vi "PDF_Interface_PDF Protokoll EPA1065_307.vi"(2 "ResultPictures":T1, 3 "PDF Optinen":T8, 4 "Deckblatt_Name":string, 5 "start":bool, 6 "SpanComponentInfos-Cluster":T7, 7 "Save PDF File Path":path, 8 "error in (no error)":errorcluster caption="Fehler (Eingang, kein Fehler)", 9 "Context (Eingang)":refnum<class "Context.lvclass">, 10 "EPA Optionsfeld":T2=enum."Rohwert", 11 "XY-Graph EPA":refnum<vi>) -> (0 "error out":errorcluster caption="Fehler (Ausgang)", 1 "Context (Ausgang)":refnum<class "Context.lvclass">)   [LabVIEW 2020, in "Linearisierung v2.lvlib" / "Protokoll.lvlib"]
uses:
  Protokoll.lvlib
  EPA Ausgabetabelle.ctl
  AktivArray.ctl
  AktivButton.ctl
  <vilib>/Simplicity AI/SAI_PDF_API/Classes/Context/Context.lvclass
  SpanEinstellungen/PDF Optionen.ctl
  SpanEinstellungen/SpanComponentInfos-Cluster.ctl
  SpanEinstellungen/ComponentInfos.ctl
  Visualisierungs Elemente/String - Ausgabefeld.ctl
  Visualisierungs Elemente/String - Eingabefeld.ctl
  EPA Optionsfeld.ctl
  PDF_Interface/PDF Interface Helper/PDFResultPictures.ctl
  Sprachverwaltung/FGV Aktion Tabelle zerlegen.ctl
  Aktion Lin Daten aufarbeiten.ctl
  EPA1065-307/Aktion FGV Auswertung sammeln.ctl
  Seiten/FT-IR/FGV FT-IR Aktionen.ctl
  Seiten/System Einstellungen V2/Aktioen FGV System Konstanten.ctl
  Seiten/FT-IR/FGV FT-IR Gasliste Aktionen.ctl
  Seiten/System Einstellungen V2/Aktion FGV SystemEinstellungenV2.ctl
  Gasteiler/Aktionen FGV Gasteiler Daten.ctl
  PDF_Interface/PDF Protokoll Standard Kopf Optionen.ctl
  PDF_Interface/PDF Interface Helper/PDFGraph.ctl
  <vilib>/Simplicity AI/SAI_PDF_API/Classes/Context/Controls/SAI_PDF_Text Align.ctl
  PDF_Interface/PDF Interface Helper/PDFCommentPosition.ctl
  PDF_Interface/PDF Interface Helper/PDFPageBreak.ctl
  <vilib>/Simplicity AI/SAI_PDF_API/Classes/Context/Controls/SAI_PDF_PDF Details.ctl
  PDF_Interface/PDF Interface Helper/PDFContentType.ctl
  PDF_Interface/PDF Interface Helper/PDFTableContentType.ctl
  PDF_Interface/PDF Interface Helper/PDFResults.ctl
  PDF_Interface/PDF Interface Helper/PDFTablePictures.ctl
  PDF_Interface/PDF Interface Helper/PDFBemerkung.ctl
  <vilib>/Simplicity AI/SAI_PDF_API/Classes/Context/Controls/SAI_PDF_Font.ctl
  <vilib>/Simplicity AI/SAI_PDF_API/Classes/Context/Controls/SAI_PDF_Font Encoding.ctl
  PDF_Interface/PDF Interface Helper/PDFTtilePageContentType.ctl
  Gasteiler/HovaCAL_Interface/Kommunikation/Aktion FGV HovaCAL Interface Autolin.ctl
  GasteilerType.ctl
  Linearisierung v2.lvlib
  EPA1065-307/Linearity verification 1065-307.lvlib
  Allgemein/allgemeine Sub-VIs.lvlib
  Seiten/FT-IR/FT-IR.lvlib
  Seiten/System Einstellungen V2/System Einstellungen V2.lvlib
  Gasteiler/Gasteiler.lvlib
  PDF_Interface/PDF Interface.lvlib
  Sprachverwaltung/Sprachverwaltung.lvlib
  PDF_Interface/PDF Interface Helper/PDF Interface Helper.lvlib
  Gasteiler/HovaCAL_Interface/Kommunikation/Kommunikation.lvlib
  SpanEinstellungen/SpanEinstellungen.lvlib
panel:
  out "Messwert:":string
  out "Serial number GT":string caption="Seriennummer:"
  out "Accuracy:":string caption="Genauigkeit:"
  out "Gas Bottle Nr.:":string caption="Gasflaschen Nr.:"
  out "Methode (Recipe):":string caption="Methode (Rezept):"
  out "Date & Time:":string caption="Datum & Zeit:"
  out "Versa Serial number:":string caption="Seriennummer:"
  out "Anlage:":string
  out "Serial number:":string caption="Seriennummer:"
  out "Messgerät:":string
  out "XY-Graph EPA":cluster{dbl[], dbl[]}[](graph) caption="XY-Graph"
  out "Aktiv":T9
  out "EPA Ausgabetabelle":T11
  out "Ergebnis:":string
  out "Konzentration:":string
  out "Komponente:":string
  out "Bearbeiter:":string
  out "Gasteiler:":string
  out "EPA Auswertung":string[][](table) caption="Evaluation"
  # "Linearity Check EPA § 1065.307"
  # "Linearity detection §1065.307"
  # "Description of the limits"
  # "Slope (a1) value between 0,99-1,01"
  # "Intercept (a0)"
  # "laboratory: Value <= 0,5% of the gas concentration"
  # "field: Value <= 1% of the gas concentration"
  # "Coefficient of determination (R²) Value >= 0,998"
  # "standard error of estimate (SEE) Value <= 1% of the gas concentration"
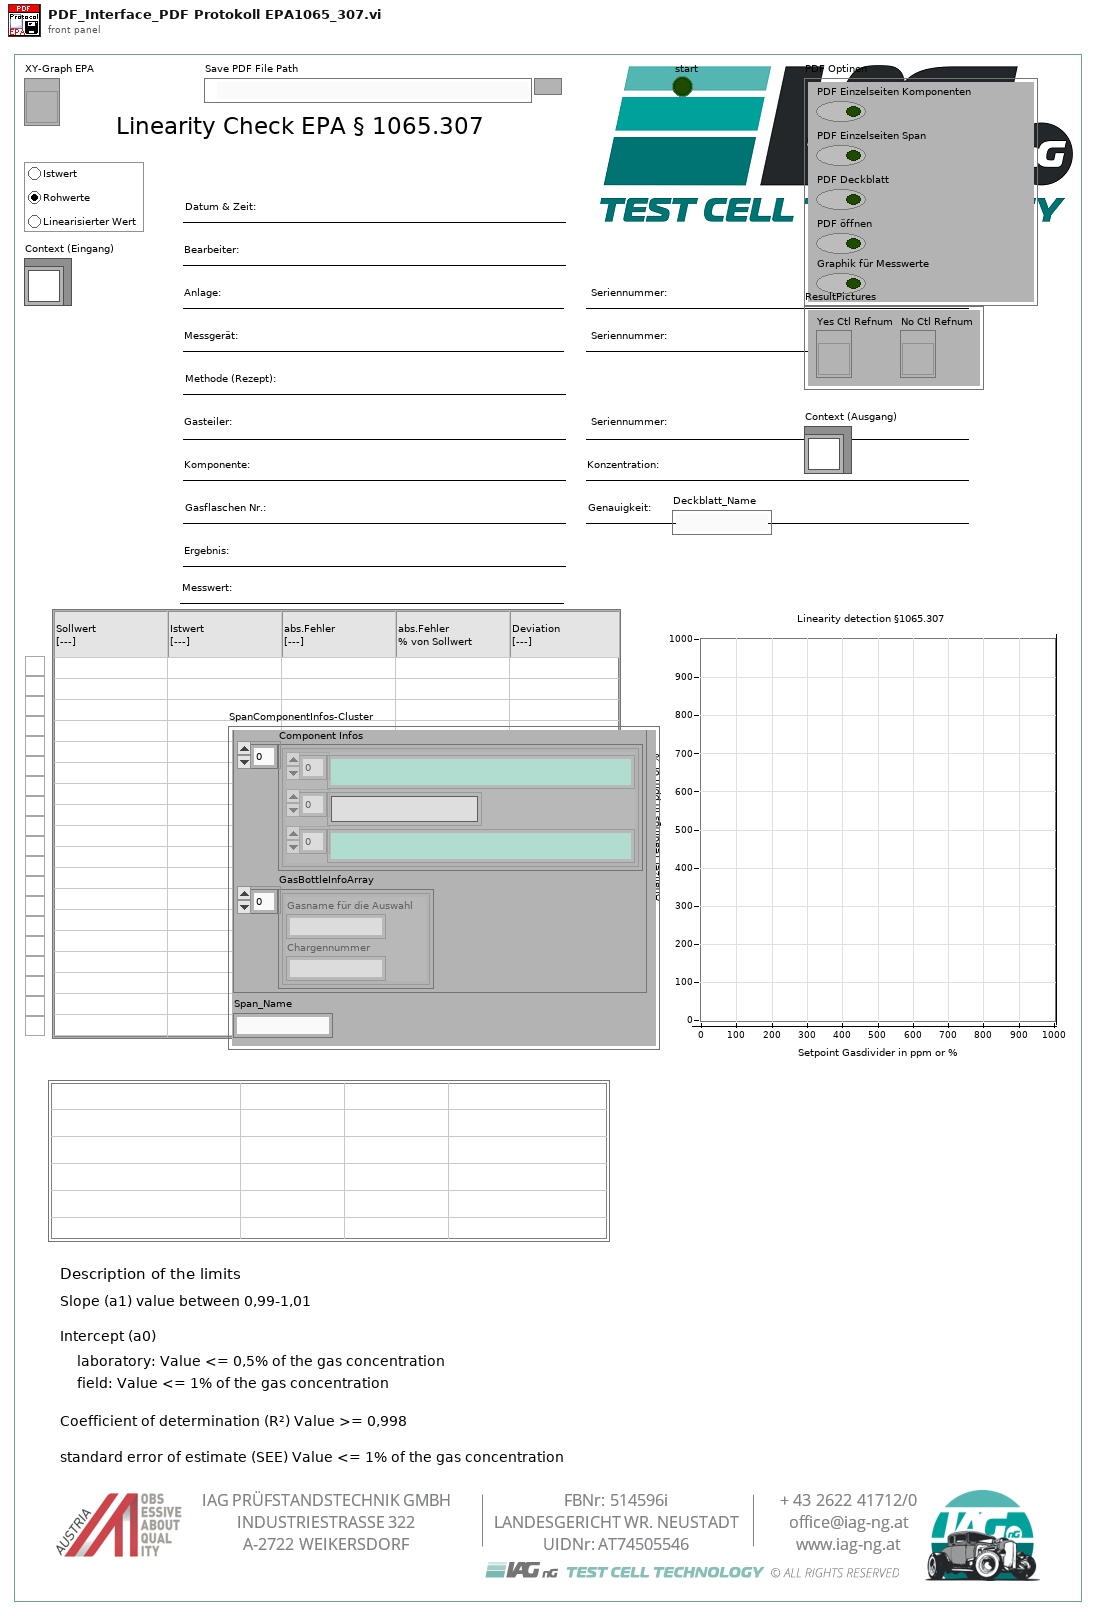
[diagram p1: front panel]
types:
  T1 = typedef "PDF Interface.lvlib/PDF Interface Helper.lvlib/PDFResultPictures.ctl" = cluster{"Yes Ctl Refnum":refnum<vi>, "No Ctl Refnum":refnum<vi>}
  T2 = typedef "Linearisierung v2.lvlib/EPA Optionsfeld.ctl" = enum32{"Istwert", "Rohwert", "Linearisierter Wert"}
  T3 = typedef "Linearisierung v2.lvlib/SpanEinstellungen.lvlib/SpanComponentInfos-Cluster.ctl" = cluster{"SPAN Names":string[], "Component Infos":T4[], "GasBottleInfoArray":cluster{"Gasname für die Auswahl":string, "Chargennummer":string}[]}
  T4 = typedef "Linearisierung v2.lvlib/SpanEinstellungen.lvlib/ComponentInfos.ctl" = cluster{T5[], T6[], T5[]}
  T5 = typedef "String - Ausgabefeld.ctl" = string
  T6 = typedef "String - Eingabefeld.ctl" = string
  T7 = cluster{"SpanComponentInfos-Cluster":T3, "Span_Name":string}
  T8 = typedef "Linearisierung v2.lvlib/SpanEinstellungen.lvlib/PDF Optionen.ctl" = cluster{"PDF Einzelseiten Komponenten":bool, "PDF Einzelseiten Span":bool, "PDF Deckblatt":bool, "PDF öffnen":bool, "Graphik für Messwerte":bool}
  T9 = typedef "Linearisierung v2.lvlib/AktivArray.ctl" = T10[]
  T10 = typedef "Linearisierung v2.lvlib/AktivButton.ctl" = bool
  T11 = typedef "Linearisierung v2.lvlib/EPA Ausgabetabelle.ctl" = string[][]
  T12 = typedef "Sprachverwaltung.lvlib/FGV Aktion Tabelle zerlegen.ctl" = enum16{"laden", "vereinzeln", "speichern"}
  T13 = typedef "PDF Interface.lvlib/PDF Protokoll Standard Kopf Optionen.ctl" = cluster{"Analysator":bool, "FT-IR Rezept":bool, "Gasteiler":bool, "Gas Komponente":bool, "Gas Flasche":bool, "LIN Protokoll":bool, "Operator":bool}
  T14 = typedef "Linearisierung v2.lvlib/Gasteiler.lvlib/Aktionen FGV Gasteiler Daten.ctl" = enum16{"lesen", "Gasteiler Daten", "Seriellen Param.", "MB-Endwert", "laden", "speichern", "Anforderung", "TCP", "Aufzeichnung Start"}
  T15 = typedef "System Einstellungen V2.lvlib/Aktion FGV SystemEinstellungenV2.ctl" = enum16{"lesen", "Analysatoren schreiben", "Analysator ändern", "Analysatoren löschen", "laden", "speichern", "Untertitel", "Analysatoren", "Neue Analysatoren", "Gasteiler schreiben", "Gasteiler ändern", "Gasteiler löschen", "Gasteiler", "Gasteiler exportieren", "Gasteiler importieren"}
  T16 = typedef "FT-IR.lvlib/FGV FT-IR Gasliste Aktionen.ctl" = enum16{"lesen", "Gasliste FT-IR", "Gasliste ausgelesen", "laden", "speichern", "löschen"}
  T17 = typedef "System Einstellungen V2.lvlib/Aktioen FGV System Konstanten.ctl" = enum16{"lesen", "laden", "speichern", "Sprache"}
  T18 = typedef "FT-IR.lvlib/FGV FT-IR Aktionen.ctl" = enum16{"lesen", "NOG setzen", "NOS setzen", "Initialisieren", "speichern", "ALLES setzen", "FT-IR Spektrum loggen", "Komm Stoppen", "Spektrum LogKonfig"}
  T19 = typedef "Linearisierung v2.lvlib/Aktion Lin Daten aufarbeiten.ctl" = enum16{"lesen", "Protkolldaten", "speichern", "laden", "EPA auswerten", "Tabelle schreiben", "Lin auswerten", "Tab init", "Stufentabelle", "EPA aktiviert", "Nachbehandlung laden", "Tabelle löschen", "Istwerte löschen", "Zeile löschen", "Zeile einfügen", "LIN aktiviert", "LIN/EPA aktiv laden", "EGAK Tab", "LIN übernehmen", "Tab init ohne Stufen"}
  T20 = typedef "Linearisierung v2.lvlib/Linearity verification 1065-307.lvlib/Aktion FGV Auswertung sammeln.ctl" = enum16{"lesen", "Auswertung", "löschen"}
  T21 = typedef "Linearisierung v2.lvlib/Gasteiler.lvlib/HovaCAL_Interface.lvlib/Kommunikation.lvlib/Aktion FGV HovaCAL Interface Autolin.ctl" = enum16{"lesen", "schreiben", "MFC Komponente fix setzen", "init"}
  T22 = typedef "PDF Interface.lvlib/PDF Interface Helper.lvlib/PDFTableContentType.ctl" = cluster{"TableHeader":string[], "Table":string[][], "Relative Column Widths (%)":sgl[], "Results":T23, "PositionBemerkung":T24, "PageBreak":T25, "TablePictures":T26, "Horizontal Align":i32}
  T23 = typedef "PDF Interface.lvlib/PDF Interface Helper.lvlib/PDFResults.ctl" = cluster{"Results":cluster{"Result Text":string, "Result":bool}[], "ResultPictures":T1, "use Pictures":bool, "Image Scale (%)":sgl, "Autoscale? (T)":bool, "Horizontal Align":i32, "Position":i32}
  T24 = typedef "PDF Interface.lvlib/PDF Interface Helper.lvlib/PDFCommentPosition.ctl" = enum16{"before", "after"}
  T25 = typedef "PDF Interface.lvlib/PDF Interface Helper.lvlib/PDFPageBreak.ctl" = enum16{"none", "before", "after", "after comment"}
  T26 = typedef "PDF Interface.lvlib/PDF Interface Helper.lvlib/PDFTablePictures.ctl" = cluster{"Ctl Refnum In":refnum<vi>[], "RowOrColumn":enum16{"Row", "Column"}, "IndexToInsert":u16, "Image Scale (%)":sgl[], "Autoscale? (T)":bool[], "Horizontal Align":i32}
  T27 = typedef "SAI_PDF_Toolkit.lvlib/Context.lvclass/SAI_PDF_Font.ctl" = cluster{"Font":string, "Size":i32, "Colour":u32, "Bold":bool, "Italic":bool, "Underline":bool, "Strikethrough":bool, "Font Encoding":T28}
  T28 = typedef "SAI_PDF_Toolkit.lvlib/Context.lvclass/SAI_PDF_Font Encoding.ctl" = enum16{"Cp1252, WinANSI", "IdentityH", "IdentityV", "Cp1250", "Cp1257", "MacRoman"}
  T29 = typedef "PDF Interface.lvlib/PDF Interface Helper.lvlib/PDFTtilePageContentType.ctl" = cluster{"Titel":string, "Header Tables":string[][][], "Bemerkungen":T30[]}
  T30 = typedef "PDF Interface.lvlib/PDF Interface Helper.lvlib/PDFBemerkung.ctl" = cluster{"Bemerkung Text":string, "Align (Left)":T31, "Add Line Feeds (F:No)":bool, "Font":T27}
  T31 = typedef "SAI_PDF_Toolkit.lvlib/Context.lvclass/SAI_PDF_Text Align.ctl" = i32
  T32 = typedef "PDF Interface.lvlib/PDF Interface Helper.lvlib/PDFGraph.ctl" = cluster{"GraphCtl Refnum":refnum<vi>, "Wrap Text (F:No)":bool, "Hide Grid (F:No)":bool, "Scale (100%)":sgl, "Align (Left)":T31, "PositionBemerkung":T24, "PageBreak":T25}
  T33 = typedef "PDF Interface.lvlib/PDF Interface Helper.lvlib/PDFContentType.ctl" = cluster{"Titel":string, "Header Table":string[][], "Table Array":T22[], "Bemerkungen":T30[]}
  T34 = typedef "SAI_PDF_Toolkit.lvlib/Context.lvclass/SAI_PDF_PDF Details.ctl" = cluster{"Title":string, "Subject":string, "Keywords":string, "Author":string, "Creator":string}
  T35 = cluster{"Header Footer Text Cluster":cluster{"Header Text":string, "Footer Text":string, "Time":string, "Page Number":string}, "PDF Details":T34}
  T36 = typedef "System Einstellungen V2.lvlib/Gasteiler.ctl" = cluster{"Gasteiler Name":string, "Gasteiler Type":string, "Gasteiler Seriennummer":string, "Gasteiler Letzte Wartung":timestamp}
  T37 = cluster{"GasteilerDefinitionsListe":T36[], "GasteilerDefinitionTextliste":string[][], "Gasteiler Strings And Values":cluster{"String":string, "Wert":string}[]}
  T38 = typedef "Linearisierung v2.lvlib/Gasteiler.lvlib/Gasteiler Daten.ctl" = cluster{"Gasteiler":T6, "Gasteiler Stufen":T39, "Gasteiler Type":T40, "Konfig Gasteiler":T41, "Gasteiler Span Eingänge":u16}
  T39 = typedef "Linearisierung v2.lvlib/Gasteiler.lvlib/Gasteiler Stufen.ctl" = u16
  T40 = typedef "Linearisierung v2.lvlib/GasteilerType.ctl" = u16
  T41 = typedef "System Einstellungen V2.lvlib/Gasteiler Auswahl.ctl" = u16
  T42 = cluster{"Modell":string, "ProjektNummer":string, "Software Version":string, "Seriennummer":string}
  T43 = typedef "Auswahlfeld.ctl" = u16
  T44 = typedef "Linearisierung v2.lvlib/Eingabetabelle.ctl" = string[][]
  T45 = typedef "Linearisierung v2.lvlib/Lin-Polynom Daten.ctl" = cluster{"Messgerät":string, "Kalibrator (Gasteiler)":string, "Bearbeiter/in":string, "Komponente":string, "Zeitstempel":timestamp, "F_max gefordert (%)":sgl, "F_max in %":sgl, "F_max in ppm":sgl, "Vorschlag Ordnung":i32, "Polynom OK":bool, "Polynomkoeff.":dbl[], "Prüfgas Konzentration":dbl, "Pfad EPA":string, "Pfad_LIN":string, "Gasnummer:":u8, "Komponentenauswahl":T46, "Verdünnungsgas":T47, "Zeitdauer Stufe":T48, "Anzahl Stufen":T48, "F_max in % EPA":sgl, "F_max in ppm EPA":sgl, "F_max in % LIN":sgl, "F_max in ppm LIN":sgl, "Punkte umkehren":bool, "EPA Optionsfeld":T2, "Autolin Hovacal":T49, "Spanfactors":sgl[], "Kalibrierauswahl":T50, "Conditions:":T51, "Gasflaschen Nr.:":string, "Bottle Accuracy":dbl, "Konfig Gasflasche":T52, "Gasflasche":T53, "HovaCAL Flow AutoLin":T54, "MFC Output":T55, "Gas Ablaufdatum":timestamp, "Lin Modus":T56, "zusätzliche Zeitdauer Erster Punkt":sgl, "Offsets":sgl[]}
  T46 = typedef "Linearisierung v2.lvlib/KomponentenArray.ctl" = cluster{"Komponente:":T43, "Konzentration":dbl}[]
  T47 = typedef "Linearisierung v2.lvlib/Gasteiler.lvlib/Prüfgas in.ctl" = u16
  T48 = typedef "Zahlen-Eingabefeld.ctl" = sgl
  T49 = typedef "Linearisierung v2.lvlib/Gasteiler.lvlib/HovaCal.lvlib/AutoLin Hovacal.ctl" = enum32{"Keine Auswahl", "Optionsauswahl 1", "Optionsauswahl 2"}
  T50 = typedef "Linearisierung v2.lvlib/Kalibrieroption.ctl" = u16
  T51 = typedef "Linearisierung v2.lvlib/Linearity verification 1065-307.lvlib/Condition.ctl" = u16
  T52 = typedef "System Einstellungen V2.lvlib/Konfig Gasflasche.ctl" = bool
  T53 = typedef "System Einstellungen V2.lvlib/Gasflasche Auswahl.ctl" = u16
  T54 = typedef "Linearisierung v2.lvlib/Gasteiler.lvlib/HovaCAL_Interface.lvlib/Controls.lvlib/Flow Einstellung.ctl" = cluster{"HovaCAL Flow Input Cluster":dbl}
  T55 = typedef "Linearisierung v2.lvlib/Gasteiler.lvlib/HovaCAL_Interface.lvlib/Controls.lvlib/Pump state.ctl" = cluster{"Run":bool}
  T56 = typedef "CalGas Aufschaltung.lvlib/Lin Modus.ctl" = u16
  T57 = cluster{"Header Size":i32, "Column Ratio left":sgl[]}
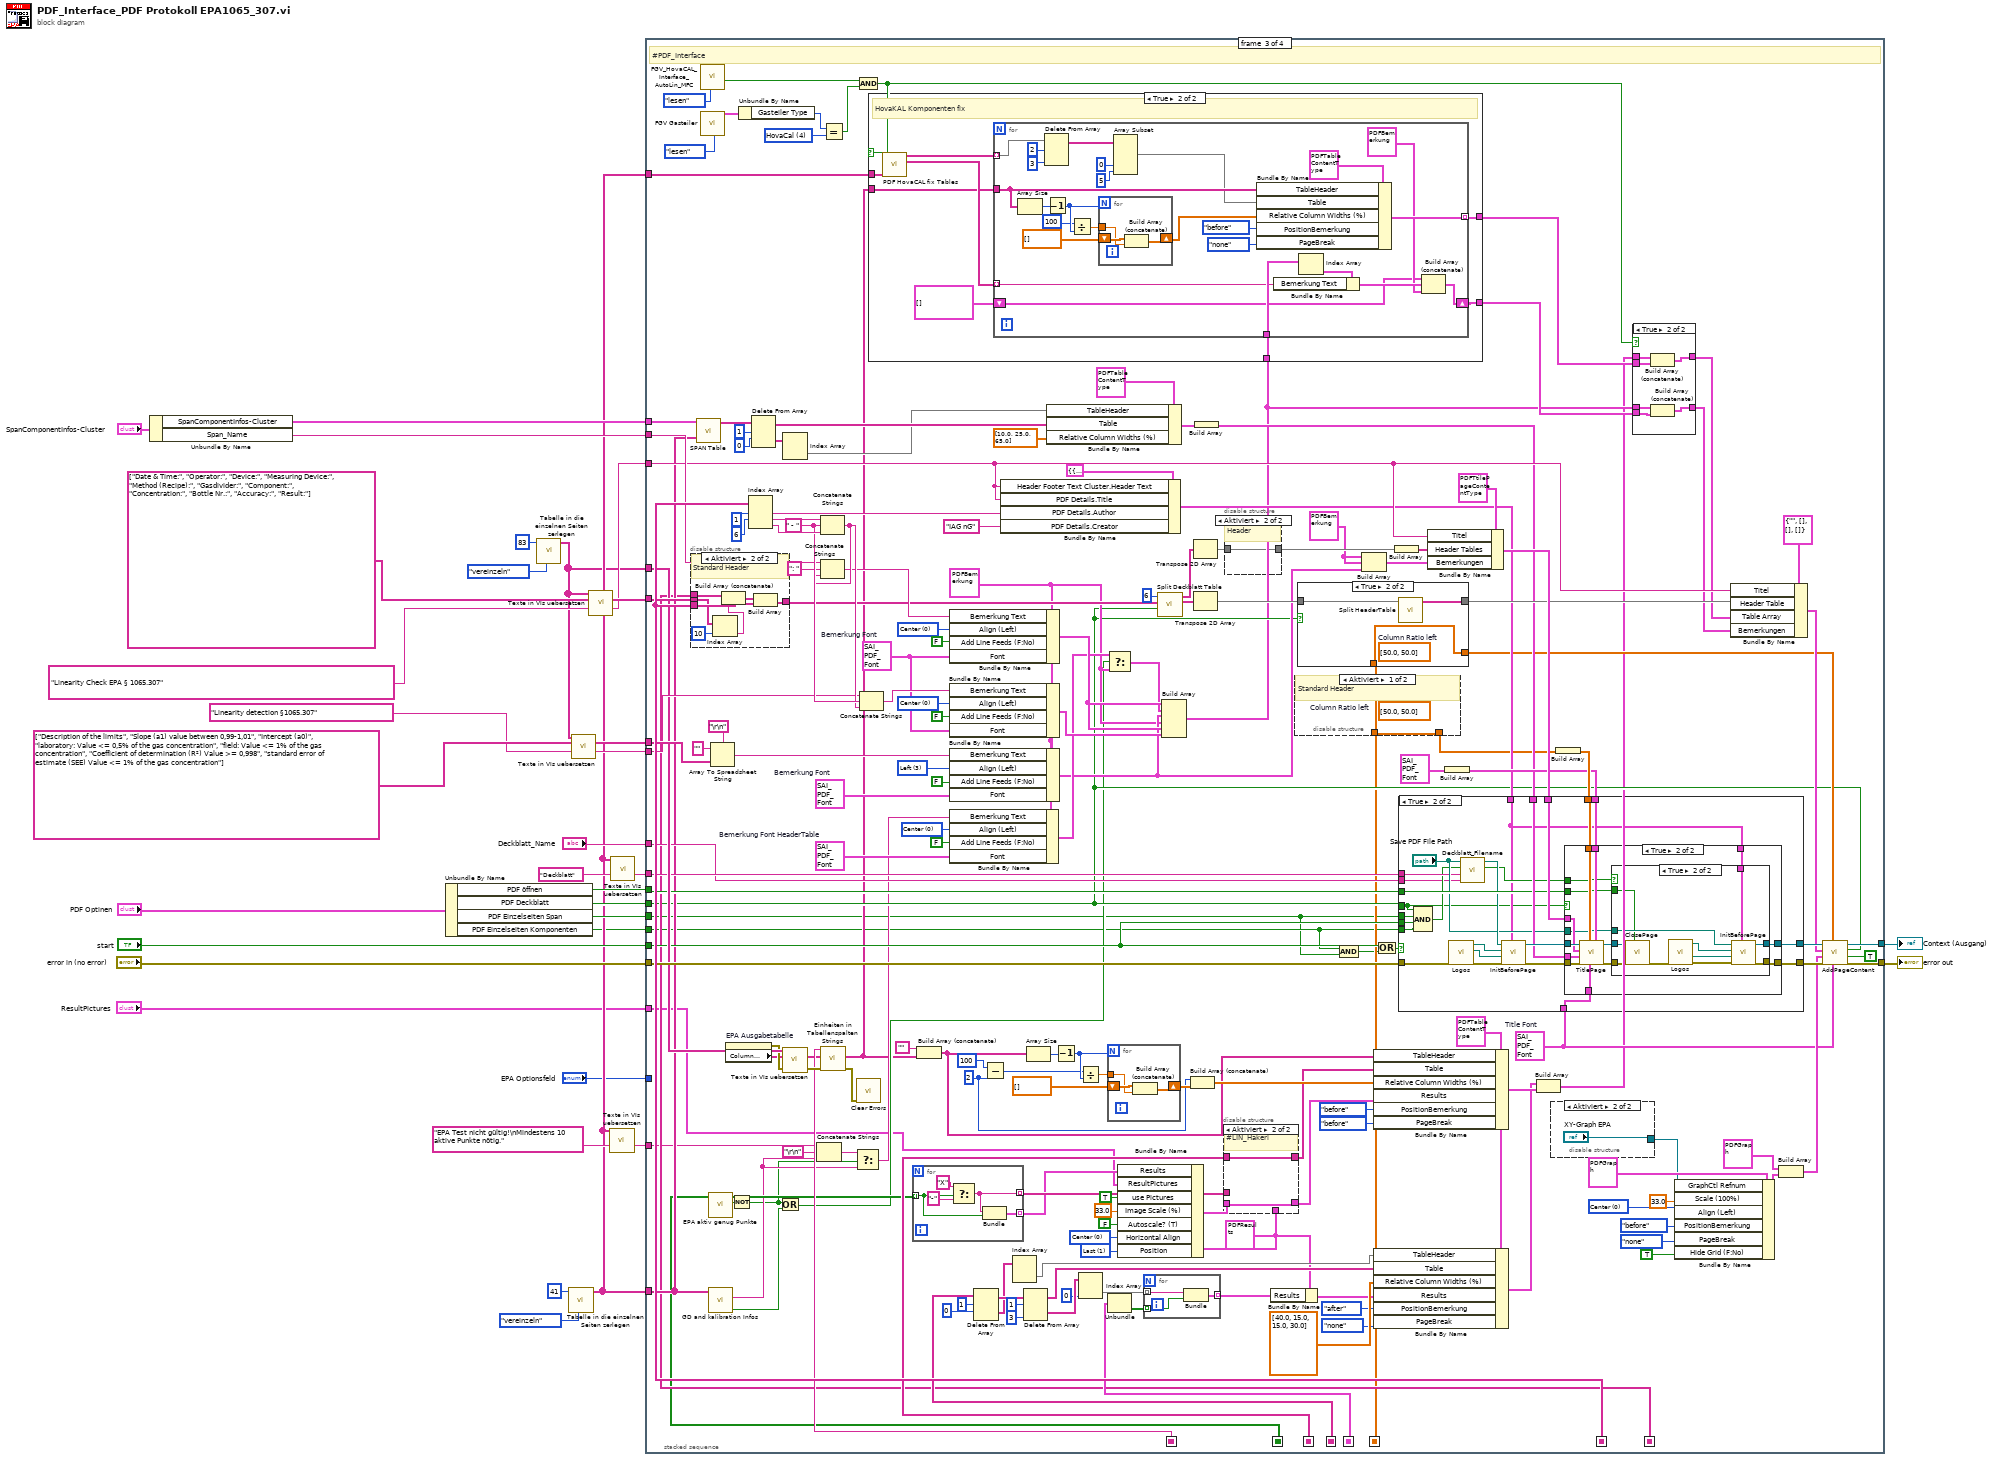
[diagram p0: block diagram]
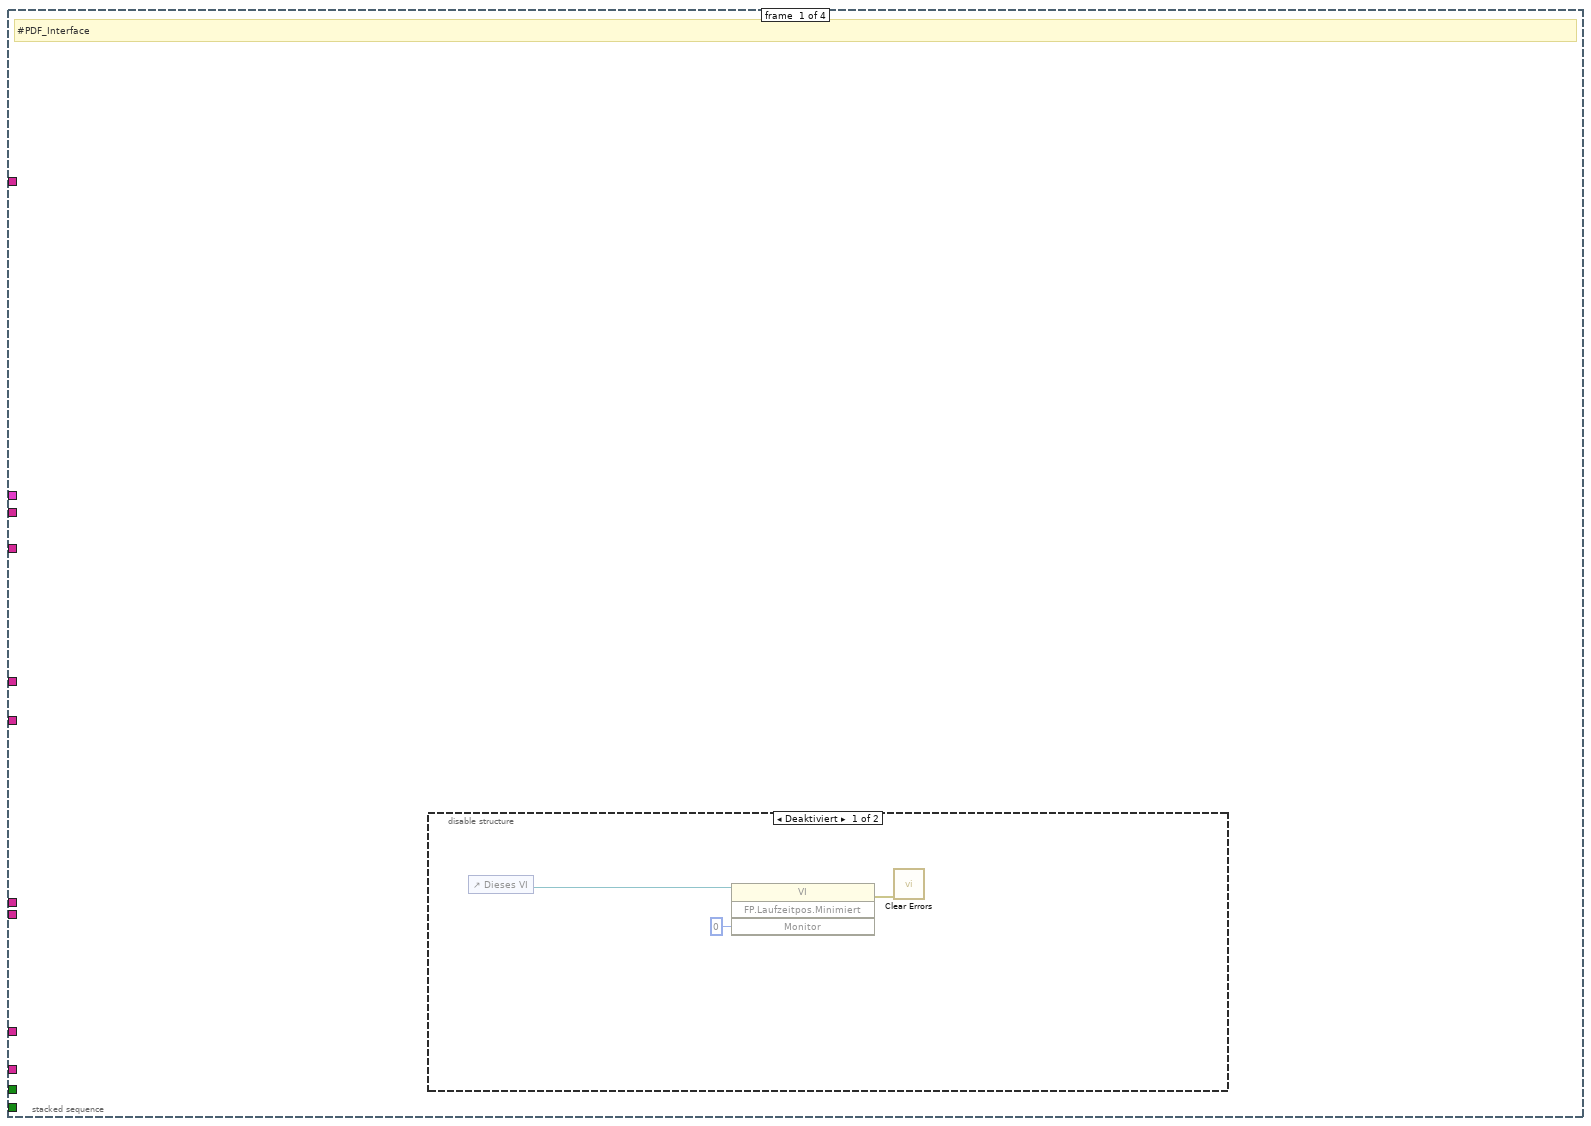
[diagram p2: hidden frame]
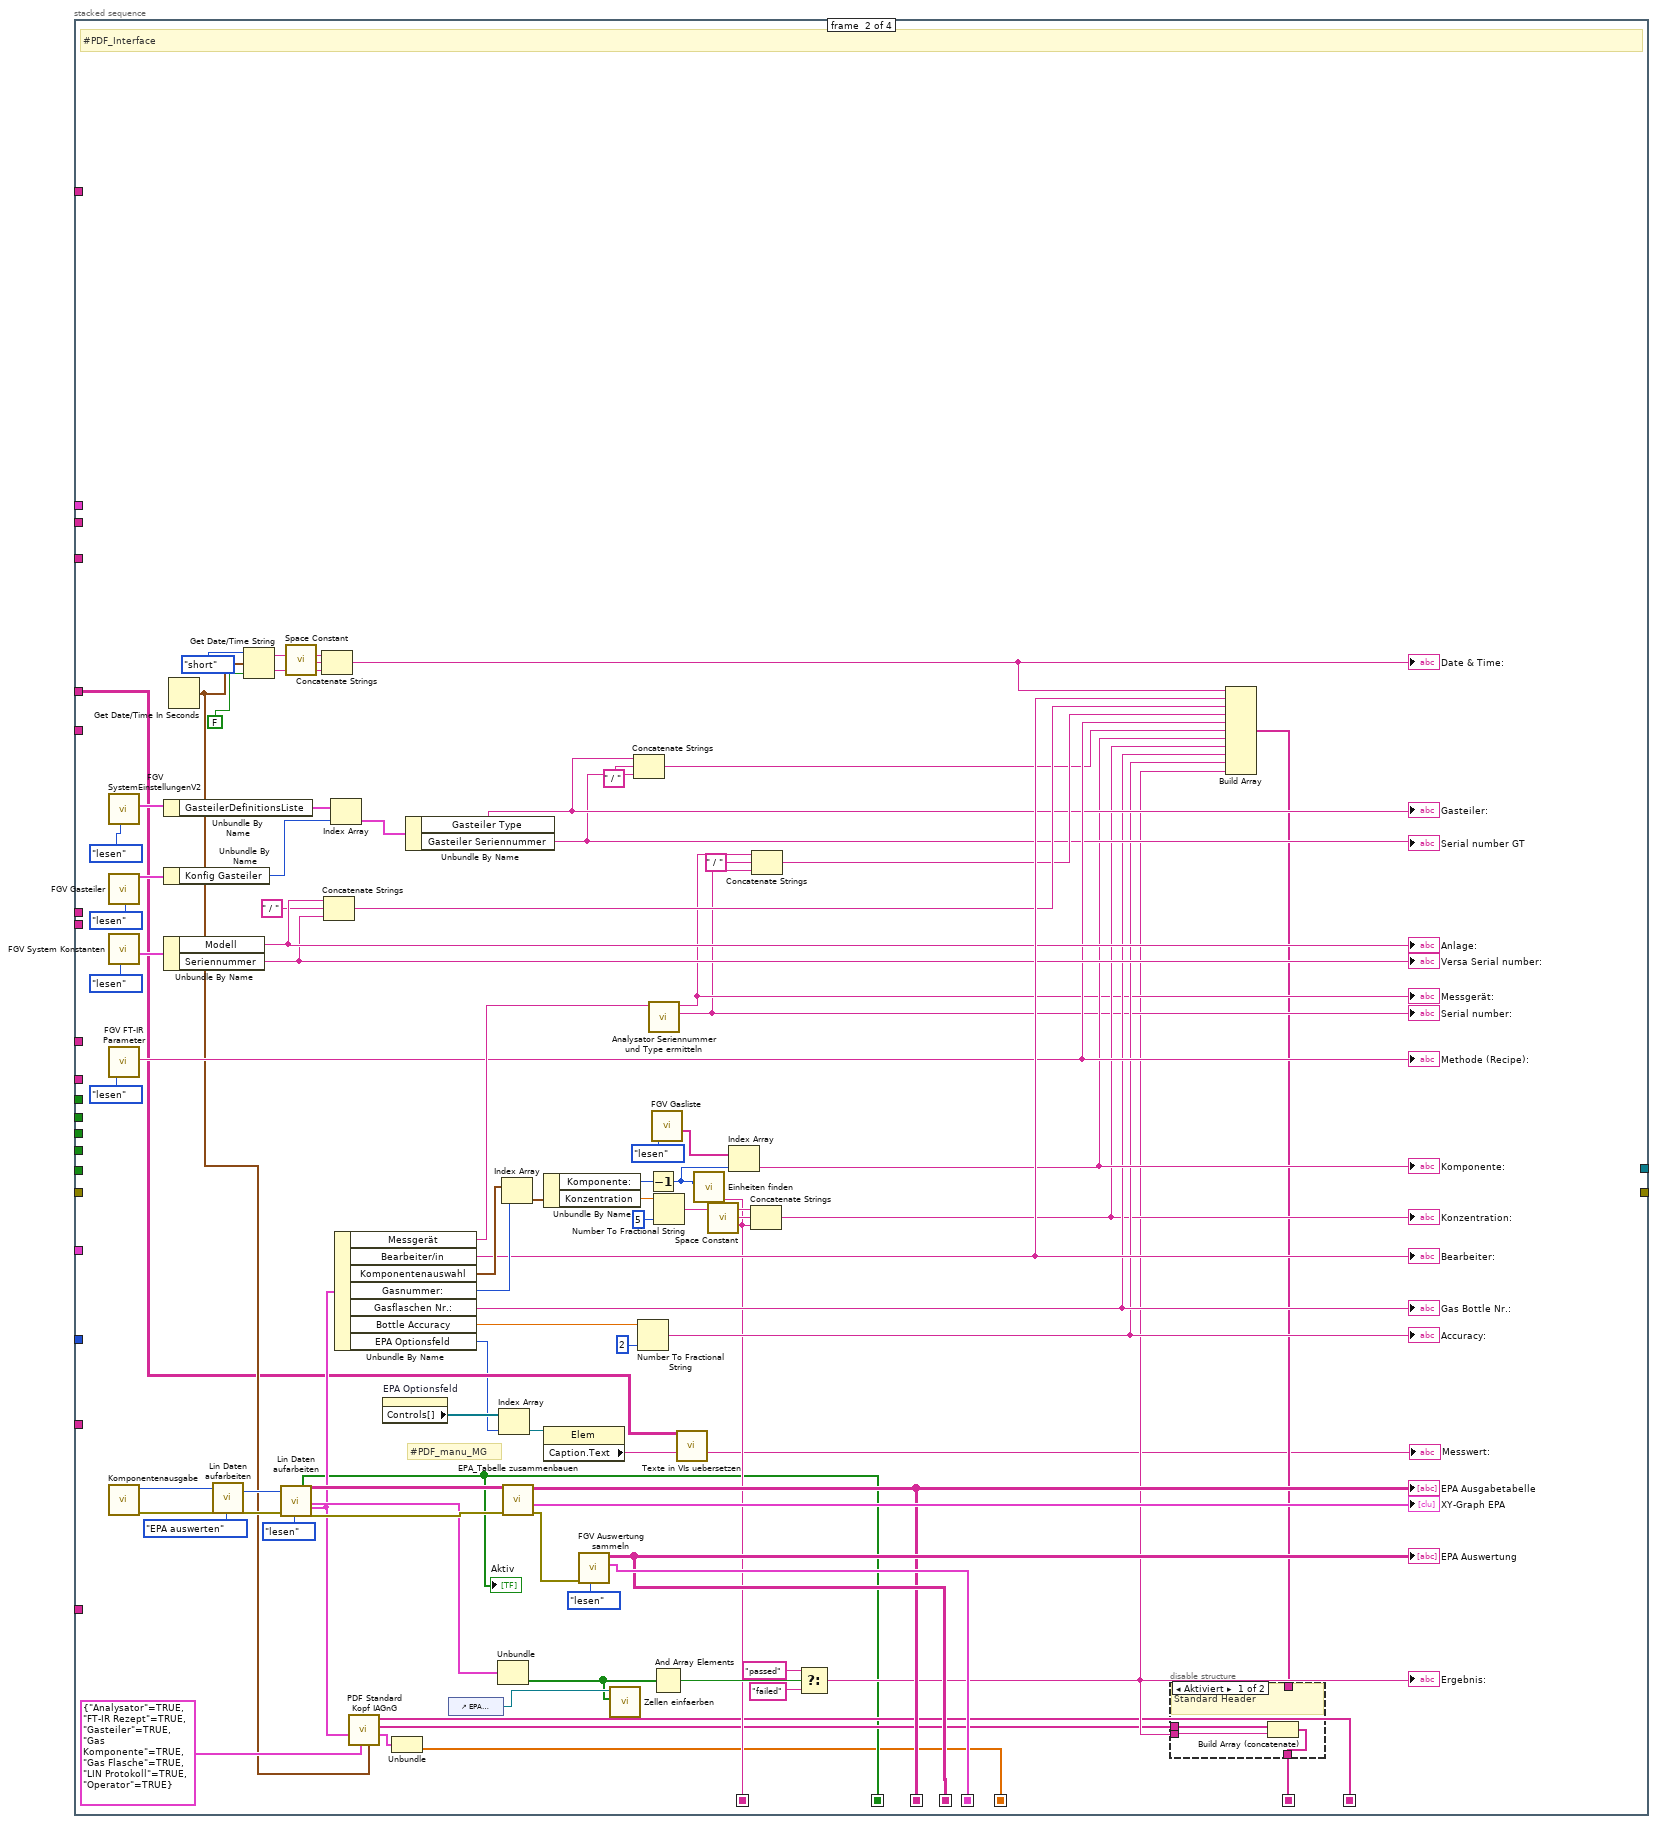
[diagram p4: hidden frame]
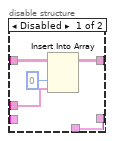
[diagram p6: hidden frame]
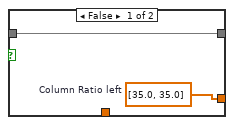
[diagram p9: hidden frame]
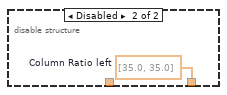
[diagram p10: hidden frame]
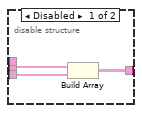
[diagram p11: hidden frame]
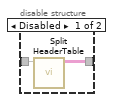
[diagram p12: hidden frame]
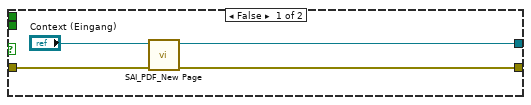
[diagram p13: hidden frame]
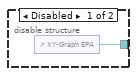
[diagram p16: hidden frame]
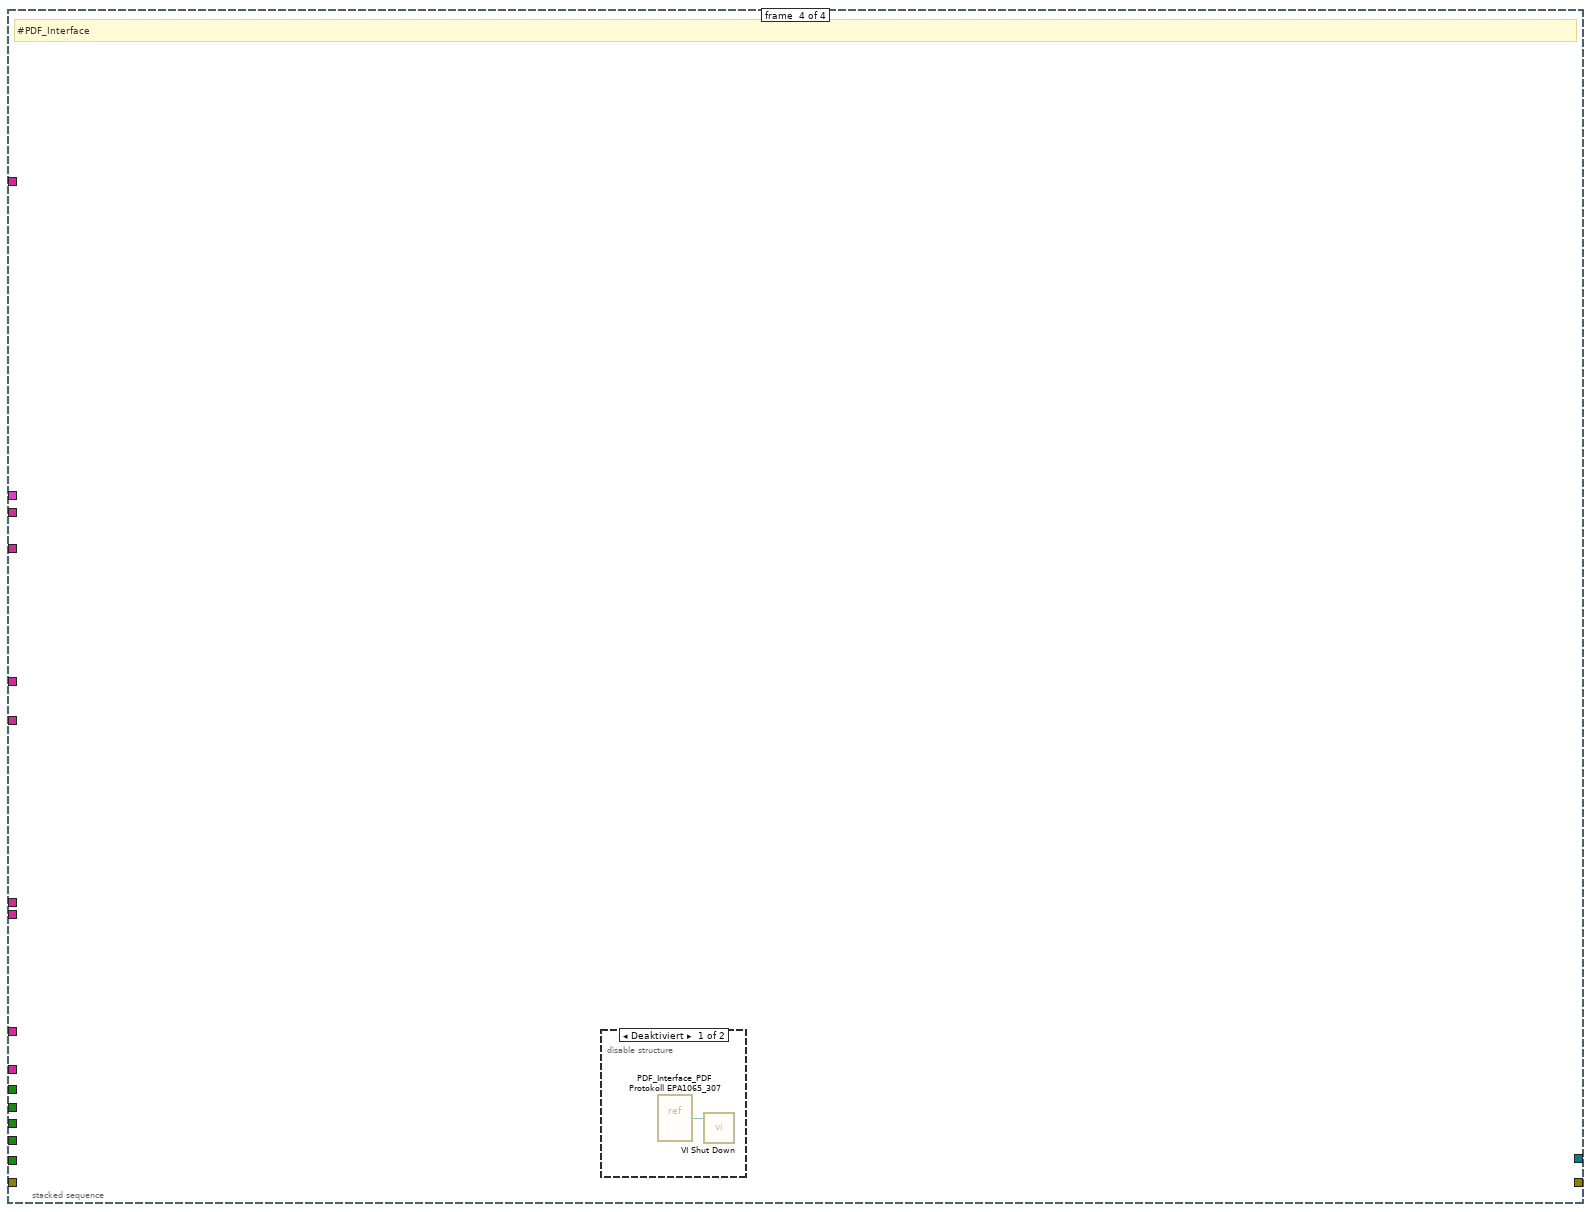
[diagram p17: hidden frame]
diagram:
  n1 = Unbundle By Name("SpanComponentInfos-Cluster") -> ("SpanComponentInfos-Cluster"=w26:T3, "Span_Name"=w29:string)
  n2 = Unbundle By Name("PDF Optinen") -> ("PDF öffnen"=w11:bool, "PDF Deckblatt"=w13:bool, "PDF Einzelseiten Span"=w12:bool, "PDF Einzelseiten Komponenten"=w2:bool)
  n3 = call "Tabelle in die einzelnen Seiten zerlegen.vi"("Aktion"=FGV_Aktion_Tabelle_zerlegen."vereinzeln", "Index (Seite)"=83) -> ("Sprachliste"=w4:string[][])  [unwired: 7 in, 2 out]
  n4 = call "Tabelle in die einzelnen Seiten zerlegen.vi"("Aktion"=FGV_Aktion_Tabelle_zerlegen."vereinzeln", "Index (Seite)"=41) -> ("Sprachliste"=w5:string[][])  [unwired: 7 in, 2 out]
  n5 = call "Texte in VIs uebersetzen.vi"("Sprachliste"=w4, "String-Array zum Übersetzen"=string[] ["Description of the limits", "Slope (a1) value between 0,99-1,01", "Intercept (a0)", "laboratory: Value <= 0,5% of the gas concentration", "field: Value <= 1% of the gas concentration", "Coefficient of determination (R²) Value >= 0,998", "standard error of estimate (SEE) Value <= 1% of the gas concentration"], "String zum Übersetzen"="Linearity detection §1065.307" ("String")) -> ("String-Array zum Übersetzen"=w17:string[], "String zum Übersetzen"=w16:string)  [unwired: 8 in, 3 out]
  n6 = call "Texte in VIs uebersetzen.vi"("Sprachliste"=w4, "String-Array zum Übersetzen"=string[] ["Date & Time:", "Operator:", "Device:", "Measuring Device:", "Method (Recipe):", "Gasdivider:", "Component:", "Concentration:", "Bottle Nr.:", "Accuracy:", "Result:"], "String zum Übersetzen"="Linearity Check EPA § 1065.307") -> ("String-Array zum Übersetzen"=w21:string[], "String zum Übersetzen"=w20:string)  [unwired: 8 in, 3 out]
  n7 = call "Texte in VIs uebersetzen.vi"("Sprachliste"=w5, "String zum Übersetzen"="EPA Test nicht gültig!\nMindestens 10 aktive Punkte nötig." ("Nachricht")) -> ("String zum Übersetzen"=w6:string)  [unwired: 9 in, 4 out]
  n8 = call "Texte in VIs uebersetzen.vi"("Sprachliste"=w5, "String zum Übersetzen"="Deckblatt") -> ("String zum Übersetzen"=w9:string)  [unwired: 9 in, 4 out]
  n9 = stacked-sequence {
    seq-local: [_ w49 _ _] -> [_ _ w296 _]
    seq-local: [_ w59 _ _] -> [_ _ w293 _]
    seq-local: [_ w64 _ _] -> [_ _ w283 _]
    seq-local: [_ w47 _ _] -> [_ _ w168 _]
    seq-local: [_ w63 _ _] -> [_ _ w281 _]
    seq-local: [_ w58 _ _] -> [_ _ w182 _]
    seq-local: [_ w48 _ _] -> [_ _ w172 _]
    seq-local: [_ w43 _ _] -> [_ _ w140 _]
    tunnel: "error in (no error)" -> [_ _ w238 _]
    tunnel: [_ _ w237 _] -> w32
    tunnel: [_ _ w236 _] -> w31
    tunnel: w29 -> [_ _ w212 _]
    tunnel: w5 -> [_ _ w174 _]
    tunnel: w26 -> [_ _ w211 _]
    tunnel: w21 -> [_ _ w198 _]
    tunnel: w20 -> [_ _ w197 _]
    tunnel: w17 -> [_ _ w196 _]
    tunnel: w16 -> [_ _ w195 _]
    tunnel: w13 -> [_ _ w169 _]
    tunnel: "start" -> [_ _ w178 _]
    tunnel: w4 -> [_ w39 w185 _]
    tunnel: w12 -> [_ _ w137 _]
    tunnel: w11 -> [_ _ w181 _]
    tunnel: w9 -> [_ _ w177 _]
    tunnel: "Deckblatt_Name" -> [_ _ w176 _]
    tunnel: w6 -> [_ _ w164 _]
    tunnel: w5 -> [_ _ w153 _]
    tunnel: "EPA Optionsfeld" -> [_ _ _ _]
    tunnel: w2 -> [_ _ w138 _]
    tunnel: "ResultPictures" -> [_ _ w132 _]
    frame #0 {
      # "#PDF_Interface"
      n10 = disable-structure shown="Deaktiviert" {
        frame Disabled {
          n11 = control-ref of="Dieses VI"() -> (w36:refnum<vi>)
          n12 = invoke class="VI" method="FP.Laufzeitpos.Minimiert"(reference=w36, "Monitor"=i16 0) -> (error out=w34:errorcluster)  [unwired: 2 in, 3 out]
          n13 = call <vilib>:"Clear Errors.vi"("error in (no error)"=w34) -> ()  [unwired: 5 in, 2 out]
        }
        frame Enabled {
        }
      }
    }
    frame #1 {
      # "#PDF_manu_MG"
      # "#PDF_Interface"
      n14 = call "FGV SystemEinstellungenV2.vi"("Aktion"=Aktion_FGV_SystemEinstellungenV2."lesen") -> ("Gasteiler"=w88:T37)  [unwired: 5 in, 5 out]
      n15 = call "FGV Gasteiler.vi"("Aktionen"=Aktionen_FGV_Gasteiler_Daten."lesen") -> ("Gasteiler Daten"=w86:T38)  [unwired: 11 in, 7 out]
      n16 = call "FGV System Konstanten.vi"("Aktionen"=Aktioen_FGV_System_Konstanten."lesen") -> ("Cluster out"=w94:T42)  [unwired: 6 in, 4 out]
      n17 = call "FGV FT-IR Parameter.vi"("Aktion"=FGV_FT-IR_Aktionen."lesen") -> ("Current Recipe"=w73:string)  [unwired: 11 in, 7 out]
      "Methode (Recipe):" <- w73
      n18 = call "Komponentenausgabe.vi"() -> ("error out"=w106:errorcluster, "Gaskomponente"=w105:T43)  [unwired: 8 in, 2 out]
      n19 = Unbundle By Name(w88) -> ("GasteilerDefinitionsListe"=w87:T36[])
      n20 = Unbundle By Name(w86) -> ("Konfig Gasteiler"=w84:T41)
      n21 = Unbundle By Name(w94) -> ("Modell"=w79:string, "Seriennummer"=w76:string)
      "Versa Serial number:" <- w76
      "Anlage:" <- w79
      n22 = Get Date/Time In Seconds() -> (seconds since 1Jan1904=w45:timestamp)
      n23 = call "Lin Daten aufarbeiten.vi"("Index (Seite)"=w105, "error in (no error)"=w106, "Aktionen"=Aktion_Lin_Daten_aufarbeiten."EPA auswerten") -> ("Index (Seite) out"=w46:i32, "error out"=w115:errorcluster)  [unwired: 14 in, 9 out]
      n24 = Get Date/Time String(date format (0)=enum16{"short", "long", "abbreviated"}."short" ("Datumsformat (0)"), seconds (now)=w45, want seconds? (F)=FALSE ("Angabe von Sekunden? (F)")) -> (date string=w98:string, time string=w99:string)
      n25 = call "Lin Daten aufarbeiten.vi"("Index (Seite)"=w46, "error in (no error)"=w115, "Aktionen"=Aktion_Lin_Daten_aufarbeiten."lesen") -> ("Aktiv EPA"=w47:T9, "Eingabetabelle"=w121:T44, "EPA Auswertung"=w111:cluster{sgl[], sgl[], bool[]}, "Lin-Polynom"=w54:T45, "error out"=w120:errorcluster)  [unwired: 14 in, 6 out]
      "Aktiv" <- w47
      n26 = call <vilib>:"Space Constant.vi"() -> ("String"=w60:string)
      n27 = Concatenate Strings(w98, w60, w99) -> (w81:string)
      "Date & Time:" <- w81
      n28 = Concatenate Strings(w79, " / " ("String"), w76) -> (w78:string)
      n29 = Index Array(array=w87, index=w84) -> (element=w83:T36)
      n30 = Unbundle By Name(w54) -> ("Messgerät"=w90:string, "Bearbeiter/in"=w80:string, "Komponentenauswahl"=w114:T46, "Gasnummer:"=w113:u8, "Gasflaschen Nr.:"=w66:string, "Bottle Accuracy"=w95:dbl, "EPA Optionsfeld"=w37:T2)
      "Bearbeiter:" <- w80
      "Gas Bottle Nr.:" <- w66
      n31 = call "PDF Standard Kopf IAGnG.vi"("Zeitstempel"=w45, "Oprtionen Cluster"=T13 {"Analysator"=TRUE, "FT-IR Rezept"=TRUE, "Gasteiler"=TRUE, "Gas Komponente"=TRUE, "Gas Flasche"=TRUE, "LIN Protokoll"=TRUE, "Operator"=TRUE}, "LIN Pototokoll-Cluster (opotional)"=w54) -> ("Size Cluster"=w44:T57, "Header Values"=w51:T5[], "Header Labels"=w48:string[])  [unwired: 5 in, 1 out]
      n32 = property on="EPA Optionsfeld" class="OptionsfelderElem (strikt)"() -> ("Controls[]"=w42:refnum<vi>[])  [unwired: 2 in, 2 out]
      n33 = Unbundle(w44) -> ("Column Ratio left"=w43:sgl[])  [unwired: 1 out]
      n34 = Unbundle By Name(w83) -> ("Gasteiler Type"=w71:string, "Gasteiler Seriennummer"=w70:string)
      "Gasteiler:" <- w71
      "Serial number GT" <- w70
      n35 = control-ref of="EPA Auswertung"() -> (w104:refnum<vi>)
      n36 = Unbundle(w111) -> (w103:bool[])  [unwired: 2 out]
      n37 = Index Array(array=w42, index=w37) -> (element=w41:refnum<vi>)
      n38 = Index Array(array=w114, index=w113) -> (element=w112:cluster{"Komponente:":T43, "Konzentration":dbl})
      n39 = call "EPA_Tabelle zusammenbauen.vi"("error in (no error)"=w120, "Eingabetabelle"=w121) -> ("error out"=w117:errorcluster, "XY-Graph"=→"XY-Graph EPA":cluster{dbl[], dbl[]}[], "EPA Ausgabetabelle"=w59:string[][])  [unwired: 7 in]
      "EPA Ausgabetabelle" <- w59
      n40 = Unbundle By Name(w112) -> ("Komponente:"=w91:T43, "Konzentration"=w108:dbl)
      n41 = property class="Elem"(reference=w41) -> ("Caption.Text"=w40:string)  [unwired: 1 in, 2 out]
      n42 = call "FGV Auswertung sammeln.vi"("Aktion"=Aktion_FGV_Auswertung_sammeln."lesen", "error in (no error)"=w117) -> ("Auswertung out"=w64:cluster{sgl[], sgl[], bool[]}, "LINVer Auswertung"=w63:string[][])  [unwired: 7 in, 1 out]
      "EPA Auswertung" <- w63
      n43 = call "Zellen einfaerben.vi"("Färben"=w103, "Tabellenref."=w104) -> ()  [unwired: 10 in]
      n44 = Concatenate Strings(w71, " / " ("String"), w70) -> (w69:string)
      n45 = Number To Fractional String(number=w95, precision (6)=i16 2 ("Genauigkeit (6)")) -> (F-format string=w65:string)  [unwired: 2 in]
      "Accuracy:" <- w65
      n46 = Decrement(x=w91) -> (x-1=w57:T43)
      n47 = call "Analysator Seriennummer und Type ermitteln.vi"("Analysator"=w90) -> ("Type"=w55:string, "Name für Protokoll"=w56:string)  [unwired: 8 in, 1 out]
      "Serial number:" <- w55
      "Messgerät:" <- w56
      n48 = call "FGV Gasliste.vi"("Aktionen"=FGV_FT-IR_Gasliste_Aktionen."lesen") -> ("Aktuelle Gasliste gesamt"=w82:T5[])  [unwired: 8 in, 2 out]
      n49 = And Array Elements(Boolean array=w103) -> (logical AND=w102:bool)
      n50 = Number To Fractional String(number=w108, precision (6)=i16 5 ("Genauigkeit (6)")) -> (F-format string=w67:string)  [unwired: 2 in]
      n51 = call "Texte in VIs uebersetzen.vi"("Sprachliste"=w39, "String zum Übersetzen"=w40) -> ("String zum Übersetzen"=→"Messwert:":string)  [unwired: 9 in, 4 out]
      n52 = call "Einheiten finden.vi"("Komponente"=w57) -> ("Einheit in String"=w58:string)  [unwired: 6 in, 4 out]
      n53 = call <vilib>:"Space Constant.vi"() -> ("String"=w61:string)
      n54 = Index Array(array=w82, index=w57) -> (element=w68:T5)
      "Komponente:" <- w68
      n55 = Concatenate Strings(w67, w61, w58) -> (w62:string)
      "Konzentration:" <- w62
      n56 = Concatenate Strings(w56, " / " ("String"), w55) -> (w74:string)
      n57 = Select(t="passed", s=w102, f="failed") -> (s? t:f=w52:string)
      "Ergebnis:" <- w52
      n58 = Build Array(w81, w80, w78, w74, w73, w69, w68, w62, w66, w65, w52) -> (w50:T5[])
      n59 = disable-structure shown="Aktiviert" {
        disable-tunnel: w52 -> [w125 _]
        disable-tunnel: w51 -> [w124 _]
        disable-tunnel: w50 -> [_ w126]
        disable-tunnel: [w123 w126] -> w49
        frame Enabled {
          # "Standard Header"
          n60 = Build Array (concatenate)(w124, w125) -> (w123:T5[])
        }
        frame Disabled {
        }
      }
    }
    frame #2 {
      w127 = 1 items=["First", "Last"] ("Position")
      w128 = T31 0 items=["Center", "Justified", "Justified All", "Left", "Right"] ("Align (Left)")
      w157 = T40 4 items=["LNI", "Analog-Display", "AVL GDU", "Horiba GDC", "HovaCal", "Horiba SGD 710C"] ("y")
      w186 = T27 {"Font"="Arial", "Size"=10, "Colour"=0, "Bold"=FALSE, "Italic"=TRUE, "Underline"=FALSE, "Strikethrough"=FALSE, "Font Encoding"=enum."Cp1252, WinANSI"}  # Bemerkung Font
      w189 = T27 {"Font"="Arial", "Size"=12, "Colour"=16711680, "Bold"=TRUE, "Italic"=TRUE, "Underline"=FALSE, "Strikethrough"=FALSE, "Font Encoding"=enum."Cp1252, WinANSI"}  # Bemerkung Font HeaderTable
      w188 = T27 {"Font"="Arial", "Size"=12, "Colour"=0, "Bold"=TRUE, "Italic"=TRUE, "Underline"=FALSE, "Strikethrough"=FALSE, "Font Encoding"=enum."Cp1252, WinANSI"}  # Bemerkung Font
      w187 = T30 {"Bemerkung Text"="", "Align (Left)"=0, "Add Line Feeds (F:No)"=FALSE, "Font"={"Font"="Arial", "Size"=10, "Colour"=0, "Bold"=FALSE, "Italic"=FALSE, "Underline"=FALSE, "Strikethrough"=FALSE, "Font Encoding"=enum."Cp1252, WinANSI"}} ("Bemerkung")
      w190 = T30 {"Bemerkung Text"="", "Align (Left)"=0, "Add Line Feeds (F:No)"=FALSE, "Font"={"Font"="Arial", "Size"=10, "Colour"=0, "Bold"=FALSE, "Italic"=FALSE, "Underline"=FALSE, "Strikethrough"=FALSE, "Font Encoding"=enum."Cp1252, WinANSI"}} ("Bemerkung")
      w133 = T23 {"Results"=[], "ResultPictures"={"Yes Ctl Refnum"=refnum, "No Ctl Refnum"=refnum}, "use Pictures"=FALSE, "Image Scale (%)"=100.0, "Autoscale? (T)"=TRUE, "Horizontal Align"=3, "Position"=0} ("Results")
      w226 = T31 0 items=["Center", "Justified", "Justified All", "Left", "Right"] ("Align (Left)")
      w224 = T27 {"Font"="Arial", "Size"=26, "Colour"=0, "Bold"=TRUE, "Italic"=FALSE, "Underline"=TRUE, "Strikethrough"=FALSE, "Font Encoding"=enum."Cp1252, WinANSI"}  # Title Font
      w241 = T31 0 items=["Center", "Justified", "Justified All", "Left", "Right"] ("Align (Left)")
      w234 = T5 " - " ("String")
      w255 = T31 0 items=["Center", "Justified", "Justified All", "Left", "Right"] ("Align (Left)")
      w269 = T31 3 items=["Center", "Justified", "Justified All", "Left", "Right"] ("Align (Left)")
      w266 = T22 {"TableHeader"=["Soll\nppm/%", "Ist\nppm/%", "Fehler\n%", "Toleranz\n%", "Ergebnis"], "Table"=[["aaa", "bbb", "ccc", "ddd"], ["111", "222", "333", "444"], ["sss", "fff", "kkk", "xxx"], ["6.5", "11.13", "19.2", "4"], ["1111", "1212", "777", "888"]], "Relative Column Widths (%)"=[22.5, 22.5, 22.5, 22.5, 4.0], "Results"={"Results"=[], "ResultPictures"={"Yes Ctl Refnum"=refnum, "No Ctl Refnum"=refnum}, "use Pictures"=FALSE, "Image Scale (%)"=100.0, "Autoscale? (T)"=TRUE, "Horizontal Align"=3, "Position"=0}, "PositionBemerkung"=enum."before", "PageBreak"=enum."before", "TablePictures"={"Ctl Refnum In"=[], "RowOrColumn"=enum."Row", "IndexToInsert"=0, "Image Scale (%)"=[], "Autoscale? (T)"=[], "Horizontal Align"=3}, "Horizontal Align"=3} ("Table Array")
      w284 = T31 0 items=["Center", "Justified", "Justified All", "Left", "Right"] ("Align (Left)")
      w285 = 2 ("y")
      # "#PDF_Interface"
      n61 = disable-structure shown="Aktiviert" {
        disable-tunnel: w296 -> [w367 w374]
        disable-tunnel: [w366 w373] -> w219
        disable-tunnel: w198 -> [w365 w371]
        disable-tunnel: w172 -> [_ w372]
        frame Disabled {
          n62 = Build Array(w365, w367) -> (w366:T5[][])
        }
        frame Enabled {
          # "Standard Header"
          n63 = Index Array(array=w371, index=10 ("Index")) -> (element=w369:string)
          n64 = Build Array (concatenate)(w372, w369) -> (w370:string[])
          n65 = Build Array(w370, w374) -> (w373:T5[][])
        }
      }
      n66 = call "SPAN Table.vi"("Sprachliste"=w174, "SpanComponentInfos-Cluster"=w211) -> ("SpanTable Info Array"=w203:string[][])  [unwired: 8 in, 1 out]
      n67 = call "FGV_HovaCAL_Interface_AutoLin_MFC.vi"("Aktion"=Aktion_FGV_HovaCAL_Interface_Autolin."lesen") -> ("fix conf"=w154:bool)  [unwired: 7 in, 3 out]
      n68 = call "FGV Gasteiler.vi"("Aktionen"=Aktionen_FGV_Gasteiler_Daten."lesen") -> ("Gasteiler Daten"=w159:T38)  [unwired: 11 in, 7 out]
      n69 = call "EPA aktiv genug Punkte.vi"("Aktiv"=w168) -> ("OK"=w165:bool, "Aktiv out"=w167:T9)  [unwired: 9 in]
      n70 = call "GD and kalibration Infos.vi"("Sprachliste"=w174) -> ("Error occured"=w173:bool, "ErrorMessage PDF"=w161:string)  [unwired: 6 in, 3 out]
      n71 = Array To Spreadsheet String(delimiter (Tab)="\r\n", array=w196, 3:"" ("Format-String")) -> (spreadsheet string=w268:string)
      n72 = property on="EPA Ausgabetabelle" class="Tbl (strikt)"() -> (error out=w184:errorcluster, "Column Headers[]"=w150:string[])  [unwired: 2 in, 1 out]
      n73 = Not(x=w165) -> (.not. x?=w141:bool)
      n74 = Unbundle By Name(w159) -> ("Gasteiler Type"=w158:T40)
      n75 = Index Array(array=w296, index #1=1 ("Index"), index #2=6 ("Index")) -> (element #1=w295:T5, element #2=w254:T5, element #3=w253:T5)  [unwired: 1 in]
      n76 = Delete From Array(array=w203, length=1 ("Länge"), index (row)=0 ("Index (Zeile)")) -> (deleted portion=w207:string[][], array with subset deleted=w208:string[][])  [unwired: 1 in]
      n77 = Or(x=w141, y=w173) -> (x .or. y?=w166:bool)
      n78 = Index Array(array=w207) -> (element=w206:string[])  [unwired: 2 in]
      n79 = call "Texte in VIs uebersetzen.vi"("Sprachliste"=w185, "String-Array zum Übersetzen"=w150) -> ("String-Array zum Übersetzen"=w152:string[])  [unwired: 9 in, 4 out]
      n80 = Concatenate Strings(w164, "\r\n", w161) -> (w162:string)
      n81 = Concatenate Strings(w254, w234, w253) -> (w230:string)
      n82 = Concatenate Strings(w212, T5 ": " ("String"), w230) -> (w229:string)
      n83 = call "Einheiten in Tabellenspalten Strings.vi"("Fehler (Eingang, kein Fehler)"=w184, "Spalten Titel mit Einheiten in"=w152, "Einheit in"=w182) -> ("Fehler (Ausgang)"=w183:errorcluster, "Spalten Titel mit Einheiten out"=w151:string[])  [unwired: 6 in, 1 out]
      n84 = Equal?(x=w158, y=w157) -> (x = y?=w155:bool)
      n85 = Select(t=w162, s=w141, f=w161) -> (s? t:f=w160:string)
      n86 = And(x=w154, y=w155) -> (x .and. y?=w142:bool)
      n87 = call <vilib>:"Clear Errors.vi"("error in (no error)"=w183) -> ()  [unwired: 5 in, 2 out]
      n88 = Concatenate Strings(w195, w234, w230) -> (w235:string)
      n89 = for {
        tunnel: w167 -> [w446] mode=indexing
        tunnel: [w447] -> w262 mode=indexing
        tunnel: [w445] -> w135 mode=indexing
        n90 = Select(t="X", s=w446, f="-") -> (s? t:f=w447:string)
        n91 = Bundle("f"=w447, "aktiv"=w446) -> (w445:cluster{"f":string, "aktiv":T10})  [unwired: 1 in]
      }
      n92 = Build Array (concatenate)("", w151) -> (w260:string[])
      n93 = Bundle By Name(cluster=w187, "Bemerkung Text"=w160, "Align (Left)"=w226, "Add Line Feeds (F:No)"=FALSE, "Font"=w189) -> (w227:T30)
      n94 = Bundle By Name(cluster=w187, "Bemerkung Text"=w229, "Align (Left)"=w255, "Add Line Feeds (F:No)"=FALSE, "Font"=w188) -> (w233:T30)
      n95 = Bundle By Name(cluster=w187, "Bemerkung Text"=w235, "Align (Left)"=w284, "Add Line Feeds (F:No)"=FALSE, "Font"=w188) -> (w240:T30)
      n96 = Bundle By Name(cluster=w187, "Bemerkung Text"=w268, "Align (Left)"=w269, "Add Line Feeds (F:No)"=FALSE, "Font"=w186) -> (w199:T30)
      n97 = Delete From Array(array=w281, length=1 ("Index (Zeile)"), index (row)=0 ("Index (Zeile)")) -> (deleted portion=w265:string[][], array with subset deleted=w279:string[][])  [unwired: 1 in]
      n98 = Subtract(x=100, y=w285) -> (x-y=w288:i32)
      n99 = Bundle By Name(cluster=T35 {"Header Footer Text Cluster"={"Header Text"="Protokoll XYZ", "Footer Text"="IAG nG", "Time"="<TIMESTAMP yyyy-MM-dd>", "Page Number"="Page <P> of <PT>"}, "PDF Details"={"Title"="Test PDF", "Subject"="Versa Tabasco", "Keywords"="", "Author"="RIW", "Creator"="IAG"}} ("Info"), "Header Footer Text Cluster.Header Text"=w197, "PDF Details.Title"=w197, "PDF Details.Author"=w295, "PDF Details.Creator"="IAG nG") -> (w175:T35)
      n100 = Index Array(array=w265) -> (element=w264:string[])  [unwired: 2 in]
      n101 = Delete From Array(array=w279, length=1 ("Länge"), index (col)=3 ("Deaktivierter Index (Spalte)")) -> (deleted portion=w258:string[][], array with subset deleted=w259:string[][])  [unwired: 1 in]
      n102 = Array Size(array=w260) -> (size(s)=w292:i32)
      n103 = Bundle By Name(cluster=T22 {"TableHeader"=[], "Table"=[], "Relative Column Widths (%)"=[], "Results"={"Results"=[], "ResultPictures"={"Yes Ctl Refnum"=refnum, "No Ctl Refnum"=refnum}, "use Pictures"=FALSE, "Image Scale (%)"=0.0, "Autoscale? (T)"=FALSE, "Horizontal Align"=0, "Position"=0}, "PositionBemerkung"=enum."after", "PageBreak"=enum."none", "TablePictures"={"Ctl Refnum In"=[], "RowOrColumn"=enum."Row", "IndexToInsert"=0, "Image Scale (%)"=[], "Autoscale? (T)"=[], "Horizontal Align"=0}, "Horizontal Align"=0} ("Table Array"), "TableHeader"=w206, "Table"=w208, "Relative Column Widths (%)"=sgl[] [10.0, 25.0, 65.0]) -> (w204:T22)
      n104 = Decrement(x=w292) -> (x-1=w291:i32)
      n105 = Divide(x=w288, y=w291) -> (x/y=w287:dbl)
      n106 = Index Array(array=w258, index (col)=0 ("Deaktivierter Index (Spalte)")) -> (element=w276:string[])  [unwired: 1 in]
      n107 = Select(t=w227, s=w166, f=w187) -> (s? t:f=w228:T30)
      n108 = for {
        N: w291 -> [_]
        shift-right: [w443] -> w286
        shift-left: sgl[] [] ("Relative Column Widths (%)") -> [w444]
        tunnel: w287 -> [w442]
        n109 = Build Array (concatenate)(w444, w442) -> (w443:dbl[])
      }
      n110 = Unbundle(w283) -> (w275:bool[])  [unwired: 2 out]
      n111 = Bundle By Name(cluster=w133, "Results"=w135, "ResultPictures"=w132, "use Pictures"=TRUE, "Image Scale (%)"=sgl 33.0, "Autoscale? (T)"=FALSE, "Horizontal Align"=w128, "Position"=w127) -> (w134:T23)
      n112 = for {
        tunnel: w276 -> [w441] mode=indexing
        tunnel: w275 -> [w440] mode=indexing
        tunnel: [w439] -> w191 mode=indexing
        n113 = Bundle("Element"=w441, w440) -> (w439:cluster{"Element":string, bool})  [unwired: 1 in]
      }
      n114 = call "Split Deckblatt Table.vi"("Deckblatt"=w169, "Array (Eingang)"=w219, "Numbre of Rows for TitlePage"=6 ("Index (Zeile)")) -> ("HeaderTable"=w217:T5[][], "TitlePage_HeaderTable"=w216:T5[][])  [unwired: 7 in]
      n115 = Build Array(w233, w228, w199, w187, w233, w240) -> (w146:T30[])
      n116 = case shown="True" w142 {
        tunnel: w151 -> [_ w322]
        tunnel: [_ w329] -> w149
        tunnel: w146 -> [_ w328]
        tunnel: [_ w327] -> w148
        tunnel: w153 -> [_ w326]
        frame False {
        }
        frame True {
          # "HovaKAL Komponenten fix"
          n117 = call "PDF HovaCAL fix Tables.vi"("Sprachliste"=w326) -> ("Bemerkungen"=w325:string[], "Eingabetabelle behandelt"=w324:string[][][])  [unwired: 9 in]
          n118 = for {
            tunnel: w322 -> [w341]
            tunnel: [w351] -> w329 mode=indexing
            tunnel: w328 -> [w344]
            tunnel: w325 -> [w342] mode=indexing
            tunnel: w324 -> [w335] mode=indexing
            shift-right: [w339] -> w327
            shift-left: T30[] [] -> [w337]
            n119 = Array Size(array=w341) -> (size(s)=w350:i32)
            n120 = Delete From Array(array=w335, length=2 ("Länge"), index (col)=3 ("Index")) -> (array with subset deleted=w333:string[][])  [unwired: 1 in, 1 out]
            n121 = Decrement(x=w350) -> (x-1=w349:i32)
            n122 = Divide(x=100, y=w349) -> (x/y=w347:dbl)
            n123 = for {
              N: w349 -> [_]
              shift-right: [w356] -> w345
              shift-left: sgl[] [] ("Relative Column Widths (%)") -> [w357]
              tunnel: w347 -> [w355]
              n124 = Build Array (concatenate)(w357, w355) -> (w356:dbl[])
            }
            n125 = Array Subset(array=w333, index (col)=0 ("Index"), length (col)=5 ("Länge")) -> (w332:string[][])  [unwired: 2 in]
            n126 = Bundle By Name(cluster=T22 {"TableHeader"=["Soll\nppm/%", "Ist\nppm/%", "Fehler\n%", "Toleranz\n%", "Ergebnis"], "Table"=[["aaa", "bbb", "ccc", "ddd"], ["111", "222", "333", "444"], ["sss", "fff", "kkk", "xxx"], ["6.5", "11.13", "19.2", "4"], ["1111", "1212", "777", "888"]], "Relative Column Widths (%)"=[22.5, 22.5, 22.5, 22.5, 4.0], "Results"={"Results"=[], "ResultPictures"={"Yes Ctl Refnum"=refnum, "No Ctl Refnum"=refnum}, "use Pictures"=FALSE, "Image Scale (%)"=100.0, "Autoscale? (T)"=TRUE, "Horizontal Align"=3, "Position"=0}, "PositionBemerkung"=enum."before", "PageBreak"=enum."before", "TablePictures"={"Ctl Refnum In"=[], "RowOrColumn"=enum."Row", "IndexToInsert"=0, "Image Scale (%)"=[], "Autoscale? (T)"=[], "Horizontal Align"=3}, "Horizontal Align"=3} ("Table Array"), "TableHeader"=w341, "Table"=w332, "Relative Column Widths (%)"=w345, "PositionBemerkung"=PDFCommentPosition."before", "PageBreak"=PDFPageBreak."none") -> (w351:T22)
            n127 = Index Array(array=w344) -> (element=w343:T30)  [unwired: 1 in]
            n128 = Bundle By Name(cluster=w343, "Bemerkung Text"=w342) -> (w340:T30)
            n129 = Build Array (concatenate)(w337, w340, T30 {"Bemerkung Text"="", "Align (Left)"=0, "Add Line Feeds (F:No)"=FALSE, "Font"={"Font"="Arial", "Size"=10, "Colour"=0, "Bold"=FALSE, "Italic"=FALSE, "Underline"=FALSE, "Strikethrough"=FALSE, "Font Encoding"=enum."Cp1252, WinANSI"}} ("Bemerkung")) -> (w339:T30[])
          }
        }
      }
      n130 = Build Array (concatenate)(w285, w286) -> (w273:dbl[])
      n131 = Transpose 2D Array(2D array=w216) -> (transposed array=w215:T5[][])
      n132 = Transpose 2D Array(2D array=w217) -> (transposed array=w239:T5[][])
      n133 = Build Array(w204) -> (w193:T22[])
      n134 = disable-structure shown="Aktiviert" {
        disable-tunnel: w293 -> [w310 w313]
        disable-tunnel: w262 -> [w309 _]
        disable-tunnel: [w308 w313] -> w261
        disable-tunnel: [w307 w312] -> w136
        disable-tunnel: w133 -> [w307 _]
        disable-tunnel: w134 -> [_ w312]
        frame Disabled {
          n135 = Insert Into Array(array=w310, index (col)=0 ("Deaktivierter Index (Spalte)"), new element=w309) -> (w308:string[][])  [unwired: 1 in]
        }
        frame Enabled {
          # "#LIN_Hakerl"
        }
      }
      n136 = disable-structure shown="Aktiviert" {
        disable-tunnel: w215 -> [w376 w377]
        disable-tunnel: [w375 w377] -> w220
        frame Disabled {
          n137 = call "Split HeaderTable.vi"("Array (Eingang)"=w376) -> ("Array (Ausgang)"=w375:T5[][])  [unwired: 10 in]
        }
        frame Enabled {
          # "Standard Header"
        }
      }
      n138 = Bundle By Name(cluster=w133, "Results"=w191) -> (w192:T23)
      n139 = disable-structure shown="Aktiviert" {
        disable-tunnel: [w363 w364] -> w171
        disable-tunnel: w140 -> [w363 _]
        frame Enabled {
          (unwired) sgl[] [50.0, 50.0]  # Column Ratio left
          # "Standard Header"
        }
        frame Disabled {
          w364 = sgl[] [35.0, 35.0]  # Column Ratio left
        }
      }
      n140 = case shown="True" w169 {
        tunnel: w239 -> [w359 w362]
        tunnel: [w359 w361] -> w221
        tunnel: [w358 w360] -> w170
        tunnel: w140 -> [_ w360]
        frame False {
          w358 = sgl[] [35.0, 35.0]  # Column Ratio left
        }
        frame True {
          (unwired) sgl[] [50.0, 50.0]  # Column Ratio left
          n141 = call "Split HeaderTable.vi"("Array (Eingang)"=w362) -> ("Array (Ausgang)"=w361:T5[][])  [unwired: 10 in]
        }
      }
      n142 = And(x=w138, y=w137) -> (x .and. y?=w139:bool)
      n143 = Build Array(w190, w190, w199) -> (w200:T30[])
      n144 = Bundle By Name(cluster=w266, "TableHeader"=w260, "Table"=w261, "Relative Column Widths (%)"=w273, "Results"=w136, "PositionBemerkung"=PDFCommentPosition."before", "PageBreak"=PDFPageBreak."before") -> (w274:T22)
      n145 = Bundle By Name(cluster=w266, "TableHeader"=w264, "Table"=w259, "Relative Column Widths (%)"=sgl[] [40.0, 15.0, 15.0, 30.0], "Results"=w192, "PositionBemerkung"=PDFCommentPosition."after", "PageBreak"=PDFPageBreak."none") -> (w267:T22)
      n146 = Or(x=w178, y=w139) -> (x .or. y?=w179:bool)
      n147 = Build Array(w220) -> (w213:T5[][][])
      n148 = Bundle By Name(cluster=T29 {"Titel"="Test mit Graph PDF", "Header Tables"=[[["Murks:", "4711"], ["HolyShit:", "0815"]]], "Bemerkungen"=[]} ("Content"), "Titel"=w197, "Header Tables"=w213, "Bemerkungen"=w200) -> (w222:T29)
      n149 = Build Array(T27 {"Font"="Arial", "Size"=10, "Colour"=0, "Bold"=FALSE, "Italic"=FALSE, "Underline"=FALSE, "Strikethrough"=FALSE, "Font Encoding"=enum."Cp1252, WinANSI"} ("HeaderTableFont")) -> (w201:T27[])
      n150 = Build Array(w267, w274) -> (w145:T22[])
      n151 = disable-structure shown="Aktiviert" {
        disable-tunnel: [w437 "XY-Graph EPA"] -> w303
        frame Disabled {
          n152 = control-ref of="XY-Graph EPA"() -> (w437:refnum<vi>)
        }
        frame Enabled {
        }
      }
      n153 = Build Array(w171) -> (w214:sgl[][])
      n154 = case shown="True" w179 {
        tunnel: [w379 w401] -> w306
        tunnel: [w380 w403] -> w305
        tunnel: w175 -> [_ w384]
        tunnel: w238 -> [w378 w388]
        tunnel: w169 -> [_ w383]
        tunnel: w224 -> [_ w400]
        tunnel: w214 -> [_ w399]
        tunnel: w222 -> [_ w398]
        tunnel: w193 -> [_ w397]
        tunnel: w201 -> [_ w396]
        tunnel: w181 -> [_ w395]
        tunnel: w177 -> [_ w392]
        tunnel: w178 -> [_ w391]
        tunnel: w137 -> [_ w390]
        tunnel: w176 -> [_ w385]
        tunnel: w138 -> [_ w382]
        frame False {
          n155 = call <vilib>:"SAI_PDF_New Page.vi"("error in"=w378, "Context In"="Context (Eingang)") -> ("error out"=w379:errorcluster, "Context Out"=w380:refnum<class "Context.lvclass">)  [unwired: 8 in]
        }
        frame True {
          n156 = Compound Arithmetic op=AND ("Mehrfacharithmetik")(w383, w390, w391, w382) -> (w389:bool)
          n157 = call "Logos.vi"("Fehler (Eingang, kein Fehler)"=w388) -> ("Fehler (Ausgang)"=w387:errorcluster, "Footer Image File Path"=w405:path, "Header Image File Path"=w406:path)  [unwired: 7 in, 1 out]
          n158 = call "Deckblatt_Filename.vi"("Deckblatt Filename"=w385, "Deckblatt Prefix"=w392, "PDF Einzelseiten & Start"=w389, "Save PDF File Path (Eingang)"="Save PDF File Path") -> ("PDF Einzelseiten & Start out"=w386:bool, "Save PDF File Path (Ausgang)"=w394:path)  [unwired: 6 in]
          n159 = call "InitBeforePage.vi"("Info"=w384, "Fehler (Eingang, kein Fehler)"=w387, "Footer Image File Path"=w405, "Header Image File Path"=w406, "Path (Dialog if Empty)"=w394) -> ("Fehler (Ausgang)"=w402:errorcluster, "Context (Ausgang)"=w404:refnum<class "Context.lvclass">)  [unwired: 5 in]
          n160 = case shown="True" w383 {
            tunnel: w404 -> [w408 w423]
            tunnel: [w408 w411] -> w403
            tunnel: w402 -> [w407 w422]
            tunnel: [w407 w410] -> w401
            tunnel: w400 -> [_ w421]
            tunnel: w399 -> [_ w420]
            tunnel: w398 -> [_ w419]
            tunnel: w397 -> [_ w418]
            tunnel: w396 -> [_ w417]
            tunnel: w386 -> [_ w416]
            tunnel: w395 -> [_ w415]
            tunnel: "Save PDF File Path" -> [_ w414]
            tunnel: w384 -> [_ w409]
            frame False {
            }
            frame True {
              n161 = call "TitlePage.vi"("HeaderTableFonts"=w417, "Title Font"=w421, "Column Ratios left"=w420, "error in"=w422, "Table Array"=w418, "Content"=w419, "Context (Eingang)"=w423) -> ("error out"=w413:errorcluster, "Context (Ausgang)"=w412:refnum<class "Context.lvclass">)  [unwired: 3 in]
              n162 = case shown="True" w416 {
                tunnel: w412 -> [w425 w436]
                tunnel: w413 -> [w424 w435]
                tunnel: [w424 w433] -> w410
                tunnel: [w425 w434] -> w411
                tunnel: w414 -> [_ w432]
                tunnel: w415 -> [_ w427]
                tunnel: w409 -> [_ w426]
                frame False {
                }
                frame True {
                  n163 = call "ClosePage.vi"("popup viewer"=w427, "Fehler (Eingang, kein Fehler)"=w435, "Context (Eingang)"=w436) -> ("Fehler (Ausgang)"=w429:errorcluster)  [unwired: 8 in]
                  n164 = call "Logos.vi"("Fehler (Eingang, kein Fehler)"=w429) -> ("Fehler (Ausgang)"=w428:errorcluster, "Footer Image File Path"=w430:path, "Header Image File Path"=w431:path)  [unwired: 7 in, 1 out]
                  n165 = call "InitBeforePage.vi"("Info"=w426, "Fehler (Eingang, kein Fehler)"=w428, "Footer Image File Path"=w430, "Header Image File Path"=w431, "Path (Dialog if Empty)"=w432) -> ("Fehler (Ausgang)"=w433:errorcluster, "Context (Ausgang)"=w434:refnum<class "Context.lvclass">)  [unwired: 5 in]
                }
              }
            }
          }
        }
      }
      n166 = case shown="True" w142 {
        tunnel: w145 -> [w314 w321]
        tunnel: [w314 w316] -> w144
        tunnel: w149 -> [_ w320]
        tunnel: w146 -> [w315 w319]
        tunnel: [w315 w318] -> w147
        tunnel: w148 -> [_ w317]
        frame False {
        }
        frame True {
          n167 = Build Array (concatenate)(w321, w320) -> (w316:T22[])
          n168 = Build Array (concatenate)(w319, w317) -> (w318:T30[])
        }
      }
      n169 = Bundle By Name(cluster=T32 {"GraphCtl Refnum"=refnum, "Wrap Text (F:No)"=FALSE, "Hide Grid (F:No)"=FALSE, "Scale (100%)"=100.0, "Align (Left)"=0, "PositionBemerkung"=enum."before", "PageBreak"=enum."after comment"} ("Graph"), "GraphCtl Refnum"=w303, "Scale (100%)"=sgl 33.0, "Align (Left)"=w241, "PositionBemerkung"=PDFCommentPosition."before", "PageBreak"=PDFPageBreak."none", "Hide Grid (F:No)"=TRUE) -> (w302:T32)
      n170 = Bundle By Name(cluster=T33 {"Titel"="", "Header Table"=[], "Table Array"=[], "Bemerkungen"=[]} ("Content"), "Titel"=w197, "Header Table"=w221, "Table Array"=w144, "Bemerkungen"=w147) -> (w299:T33)
      n171 = Build Array(T32 {"GraphCtl Refnum"=refnum, "Wrap Text (F:No)"=FALSE, "Hide Grid (F:No)"=FALSE, "Scale (100%)"=0.0, "Align (Left)"=0, "PositionBemerkung"=enum."before", "PageBreak"=enum."after comment"} ("Element"), w302) -> (w272:T32[])
      n172 = call "AddPageContent.vi"("Graph last"=TRUE, "Deckblatt"=w169, "Title Font"=w224, "Column Ratio left"=w170, "error in"=w306, "Graph Array"=w272, "Content"=w299, "Context (Eingang)"=w305) -> ("error out"=w237:errorcluster, "Context (Ausgang)"=w236:refnum<class "Context.lvclass">)  [unwired: 2 in]
    }
    frame #3 {
      # "#PDF_Interface"
      n173 = disable-structure shown="Deaktiviert" {
        frame Disabled {
          n174 = vi-ref "PDF_Interface_PDF Protokoll EPA1065_307.vi"() -> (w450:refnum<vi>)
          n175 = call "VI Shut Down.vi"("VI Referenz"=w450) -> ()  [unwired: 11 in]
        }
        frame Enabled {
        }
      }
    }
  }
  "error out" <- w32
  "Context (Ausgang)" <- w31
